vi "_ModeMgr.Test.vi"() -> ()   [LabVIEW 2018]
uses:
  ModeMgr.Mode Settings.ctl
  Mode Manager.lvclass
panel:
  out "Mode Settings":T1[](array[typedef])
  out "Mode":string
  in  "Init":bool
  in  "stop":bool
  out "error out":errorcluster
  in  "Get Mode":bool
  in  "Mode Config Path":path=path "C:/MTE/Facility/Modes.json"
  in  "Mode Control":u16(ring) items=["Production", "Technician", "Engineering"]
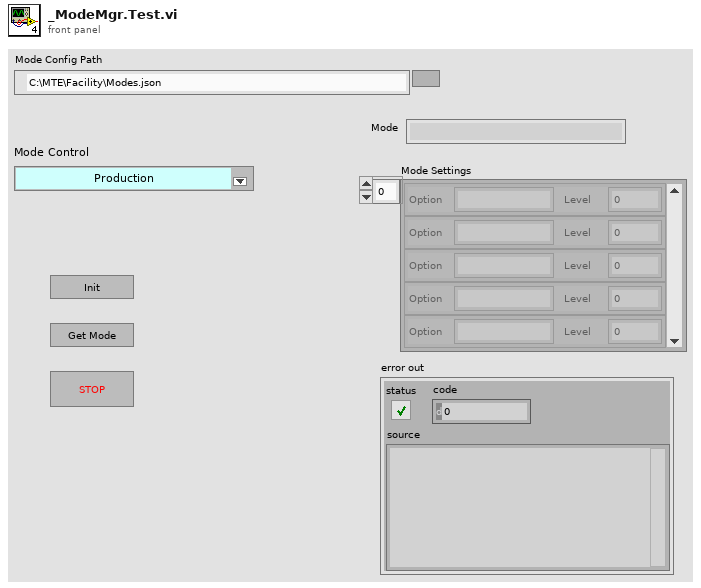
[diagram p1: front panel]
types:
  T1 = typedef "ModeMgr.Mode Settings.ctl" = cluster{"Option":string, "Level":i32}
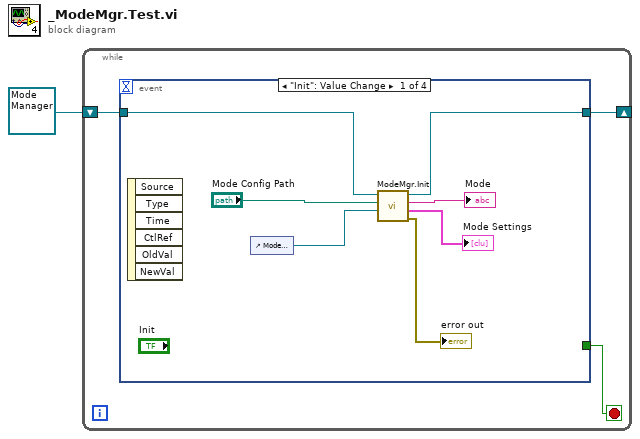
[diagram p0: block diagram]
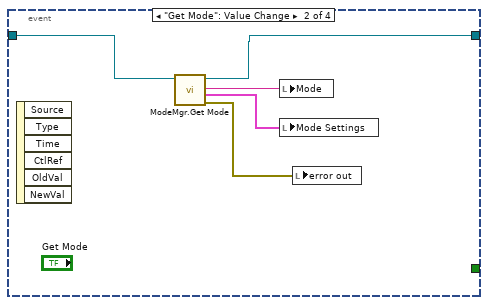
[diagram p2: hidden frame]
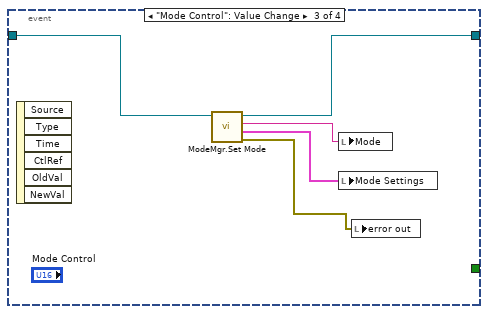
[diagram p3: hidden frame]
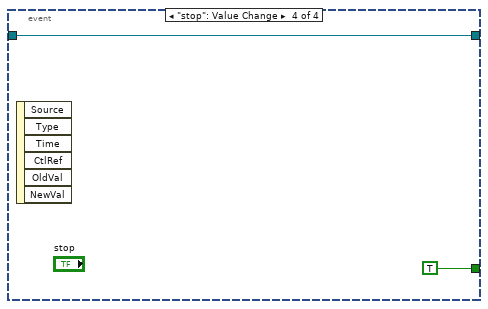
[diagram p4: hidden frame]
diagram:
  n1 = while {
    shift-right: [w3] -> _
    shift-left: refnum<class "Mode Manager.lvclass"> refnum ("Mode Manager.lvclass") -> [w4]
    stop <- w2 stop-if-true
    n2 = event shown="[0] \"Init\": Value Change" {
      selector: _ -> [_ _ _ _]
      dyn-events: _ -> [_ _ _ _]
      timeout: _ -> [_ _ _ _]
      tunnel: w4 -> [w11 w16 w21 w22]
      tunnel: [w9 w15 w20 w22] -> w3
      tunnel: [_ _ _ TRUE] -> w2
      event "Init": Value Change {
        n3 = event-data() -> ()  [unwired: 1 in, 6 out]
        n4 = control-ref of="Mode Control"() -> (w6:refnum<vi>)
        n5 = call "ModeMgr.Init.vi"("ControlRef"=w6, "Config File"="Mode Config Path", "ModeMgr In"=w11) -> ("error out"=→"error out":errorcluster, "Mode Settings"=→"Mode Settings":T1[], "Mode"=→"Mode":string, "ModeMgr Out"=w9:refnum<class "Mode Manager.lvclass">)  [unwired: 5 in]
      }
      event "Get Mode": Value Change {
        n6 = event-data() -> ()  [unwired: 1 in, 6 out]
        n7 = call "ModeMgr.Get Mode.vi"("ModeMgr In"=w16) -> ("error out"=w12:errorcluster, "Settings"=w13:T1[], "Mode"=w14:string, "ModeMgr Out"=w15:refnum<class "Mode Manager.lvclass">)  [unwired: 7 in]
        n8 = local write "Mode"(w14) -> ()
        n9 = local write "Mode Settings"(w13) -> ()
        n10 = local write "error out"(w12) -> ()
      }
      event "Mode Control": Value Change {
        n11 = event-data() -> ()  [unwired: 1 in, 6 out]
        n12 = call "ModeMgr.Set Mode.vi"("ModeMgr In"=w21) -> ("error out"=w17:errorcluster, "Settings"=w18:T1[], "Mode"=w19:string, "ModeMgr Out"=w20:refnum<class "Mode Manager.lvclass">)  [unwired: 6 in, 1 out]
        n13 = local write "Mode"(w19) -> ()
        n14 = local write "Mode Settings"(w18) -> ()
        n15 = local write "error out"(w17) -> ()
      }
      event "stop": Value Change {
        n16 = event-data() -> ()  [unwired: 1 in, 6 out]
      }
    }
  }
